vi "to_variant_MOVE_SYSTEM_cmd_data.vi"(10 "move info array":T1[](array[typedef]), 11 "MotorSystem.lvclass":refnum<class "MotorSystem.lvclass">) -> (3 "variant":variant)   [LabVIEW 2016, in "MotionControl.lvlib"]
uses:
  <userlib>/MotionControl/MotionControl.lvlib
  <userlib>/MotionControl/MotorSystem/SavedDimensionCluster.ctl
  <userlib>/MotionControl/OneMotion/unit mode.ctl
  <userlib>/MotionControl/MotorSystem/MotorSystem.lvclass
  <userlib>/MotionControl/OneMotion/OneMotion.lvclass
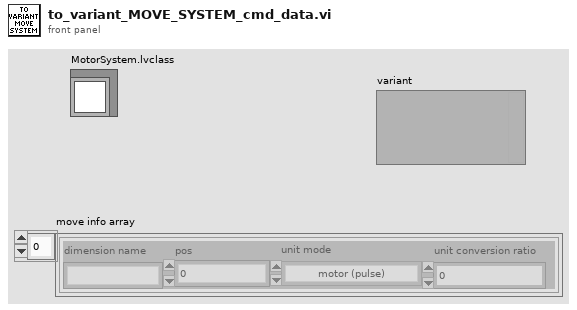
[diagram p1: front panel]
types:
  T1 = typedef "MotionControl.lvlib/MotorSystem.lvclass/SavedDimensionCluster.ctl" = cluster{"dimension name":string, "pos":dbl, "unit mode":T2, "unit conversion ratio":dbl}
  T2 = typedef "MotionControl.lvlib/OneMotion.lvclass/unit mode.ctl" = enum16{"motor (pulse)", "linear (mm) or radial (degree)"}
  T3 = cluster{"MotorSystem.lvclass":refnum<class "MotorSystem.lvclass">, "move info array":T1[]}
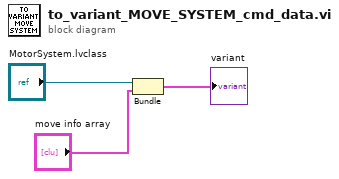
[diagram p0: block diagram]
diagram:
  n1 = Bundle("MotorSystem.lvclass"="MotorSystem.lvclass", "move info array"="move info array") -> (→"variant":T3)  [unwired: 1 in]
